vi "Start Live Mode.vi"(8 "error in (no error)":errorcluster, 10 "Camera Settings":T1={"Exposure Time (ms)"=100.0, "Binning"=enum."2x2", "Scan Mode"=0, "Frames to Acquire"=1000.0, "Pixel Correction"=FALSE, "Frames to Skip"=0, "File Path"=path "", "Duty cycle"=0.0, "ALEX"=FALSE, "Shutter Enable"=[], "fluidics trigger frame"=0, "Bit Depth"=0, "Image Width (px)"=0, "Image Height (px)"=0, "Horizontal Offset (px)"=0, "Vertical Offset (px)"=0} {"fluidics trigger frame" max=60000 step=1; "Exposure Time (ms)" min=1.0 max=10000.0 step=1.0}, 11 "Andor Camera in":refnum<class "Andor Camera.lvclass">) -> (0 "error out":errorcluster, 3 "Andor Camera out":refnum<class "Andor Camera.lvclass">)   [LabVIEW 2018, in "Andor Camera.lvlib" / "Andor Camera.lvclass"]
uses:
  Andor Camera.lvclass
  Resources/Type Defs/Camera Settings.ctl
  <userlib>/atmcd64d.llb/AcquisitionMode_mode typedef.ctl
  Camera/Camera.lvclass
panel:
  out "DLL error code 2":u32
  out "DLL error code":u32
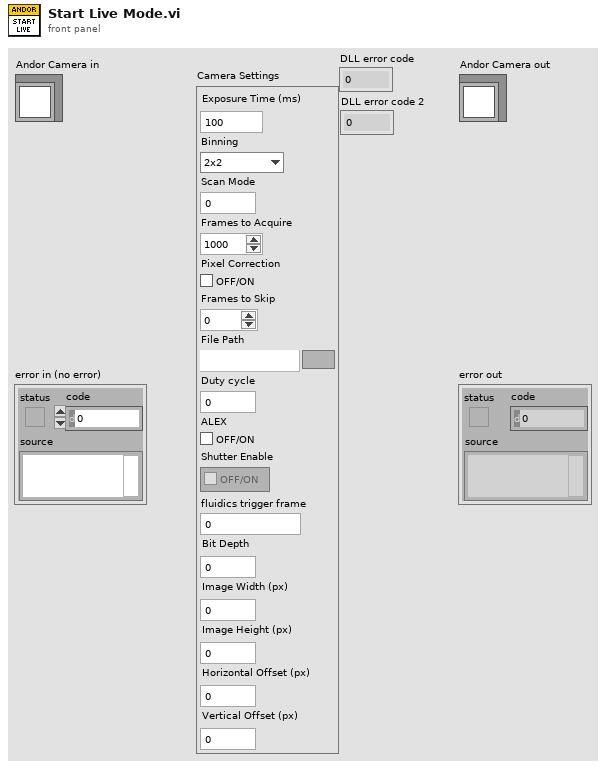
[diagram p1: front panel]
types:
  T1 = typedef "Camera Settings.ctl" = cluster{"Exposure Time (ms)":dbl, "Binning":enum16{"1x1", "2x2", "4x4"}, "Scan Mode":i32, "Frames to Acquire":dbl, "Pixel Correction":bool, "Frames to Skip":u32, "File Path":path, "Duty cycle":dbl, "ALEX":bool, "Shutter Enable":bool[], "fluidics trigger frame":u16, "Bit Depth":u16, "Image Width (px)":u16, "Image Height (px)":u16, "Horizontal Offset (px)":u16, "Vertical Offset (px)":u16}
  T2 = typedef "AcquisitionMode_mode typedef.ctl" = enum16{"Reserved (0)", "Single Scan", "Accumulate", "Kinetics", "Fast Kinetics", "Run Till Abort", "Reserved (6)", "Reserved (7)", "Reserved (8)", "Time Delayed Integration"}
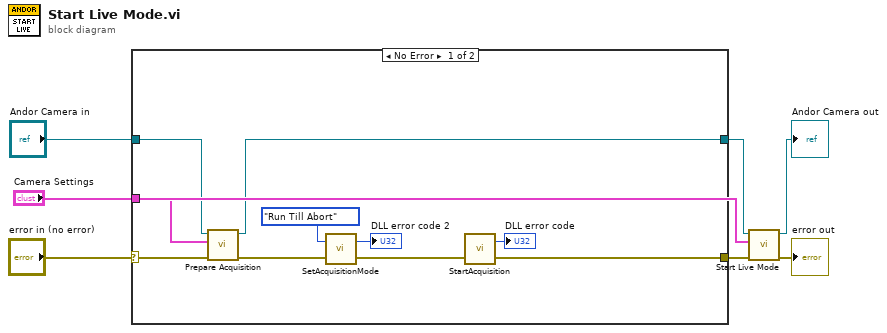
[diagram p0: block diagram]
diagram:
  n1 = case shown="No Error" "error in (no error)" {
    selector: "error in (no error)" -> [w15 w18]
    tunnel: "Andor Camera in" -> [w17 w19]
    tunnel: [w16 w19] -> w4
    tunnel: [w12 w18] -> w2
    tunnel: "Camera Settings" -> [w11 _]
    frame No Error {
      n2 = call-dynamic "Prepare Acquisition.vi"("error in (no error)"=w15, "Camera Settings"=w11, "Andor Camera in"=w17) -> ("error out"=w14:errorcluster, "Andor Camera out"=w16:refnum<class "Andor Camera.lvclass">)  [unwired: 7 in]
      n3 = call <userlib>:"SetAcquisitionMode.vi"("error in (no error)"=w14, "mode"=AcquisitionMode_mode_typedef."Run Till Abort") -> ("error out"=w13:errorcluster, "DLL error code"=→"DLL error code 2":u32)
      n4 = call <userlib>:"StartAcquisition.vi"("error in (no error)"=w13) -> ("error out"=w12:errorcluster, "DLL error code"=→"DLL error code":u32)  [unwired: 1 in]
    }
    frame Error {
    }
  }
  n5 = call-parent "Start Live Mode.vi"("error in (no error)"=w2, "Camera Settings"="Camera Settings", "Camera in"=w4) -> ("error out"=→"error out":errorcluster, "Camera out"=→"Andor Camera out":refnum<class "Andor Camera.lvclass">)  [unwired: 7 in]
